vi "RIO_Neunet.vi"() -> ()   [LabVIEW 2015]
panel:
  in  "Stop":bool
  out "Received Data":dbl(graph)
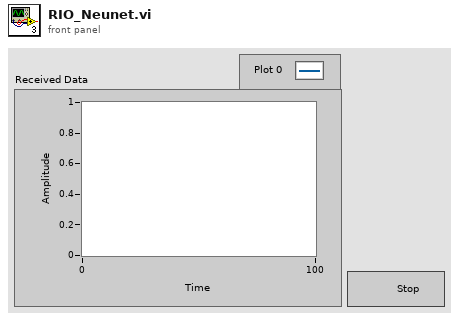
[diagram p1: front panel]
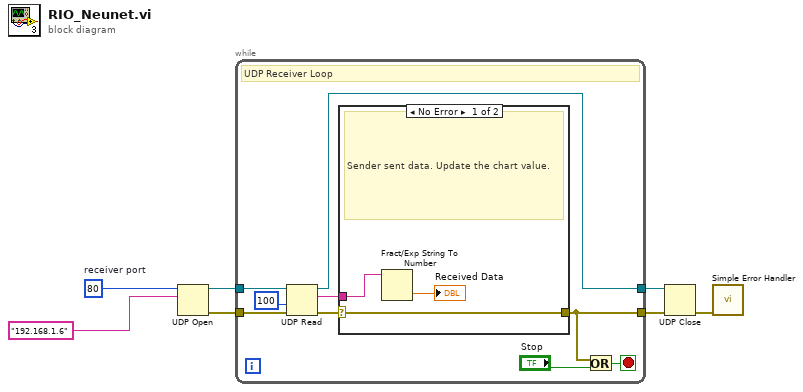
[diagram p0: block diagram]
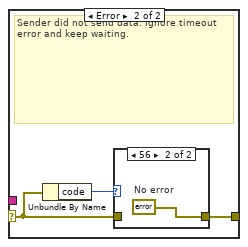
[diagram p2: hidden frame]
diagram:
  w2 = u16 80  # receiver port
  n1 = UDP Open(10:"192.168.1.6" ("service name"), 11:w2) -> (port=w3:refnum<k16>, 0:w4:errorcluster)  [unwired: 3 in, 1 out]
  n2 = while {
    tunnel: w3 -> [w16]
    tunnel: [w8] -> w7
    tunnel: w4 -> [w13]
    tunnel: [w9] -> w5
    stop <- w14 stop-if-true
    # "UDP Receiver Loop"
    n3 = UDP Read(connection ID=w16, timeout ms (25000)=100, 8:w13) -> (data out=w11:string, error out=w10:errorcluster, 3:w8:refnum<k16>)  [unwired: 3 out]
    n4 = case shown="No Error" w10 {
      selector: w10 -> [w17 w21]
      tunnel: w11 -> [w19 _]
      tunnel: [w17 w20] -> w9
      frame No Error {
        # "Sender sent data. Update the chart value."
        n5 = Fract/Exp String To Number(string=w19) -> (number=→"Received Data":dbl)  [unwired: 3 in, 1 out]
      }
      frame Error {
        # "Sender did not send data. Ignore timeout error and keep waiting."
        n6 = Unbundle By Name(w21) -> ("code"=w22:i32)
        n7 = case shown="56" w22 {
          tunnel: w21 -> [w23 _]
          tunnel: [w23 w24] -> w20
          frame Default {
          }
          frame 56 {
            w24 = errorcluster {"status"=FALSE, "code"=0, "source"=""}  # No error
          }
        }
      }
    }
    n8 = Or(x=w9, y="Stop") -> (x .or. y?=w14:bool)
  }
  n9 = UDP Close(connection ID=w7, 8:w5) -> (error out=w6:errorcluster)  [unwired: 1 out]
  n10 = call <vilib>:"Simple Error Handler.vi"("error in (no error)"=w6) -> ()  [unwired: 1 in, 8 out]
